vi "dc voltmeter.vi"() -> ()   [LabVIEW 2015]
panel:
  out "Color Indicator":u32(colorbox)
  out "String":string
  in  "Voltage":dbl
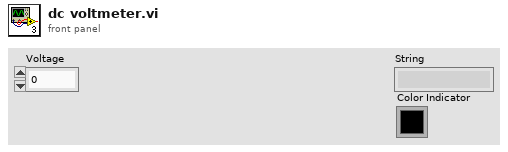
[diagram p1: front panel]
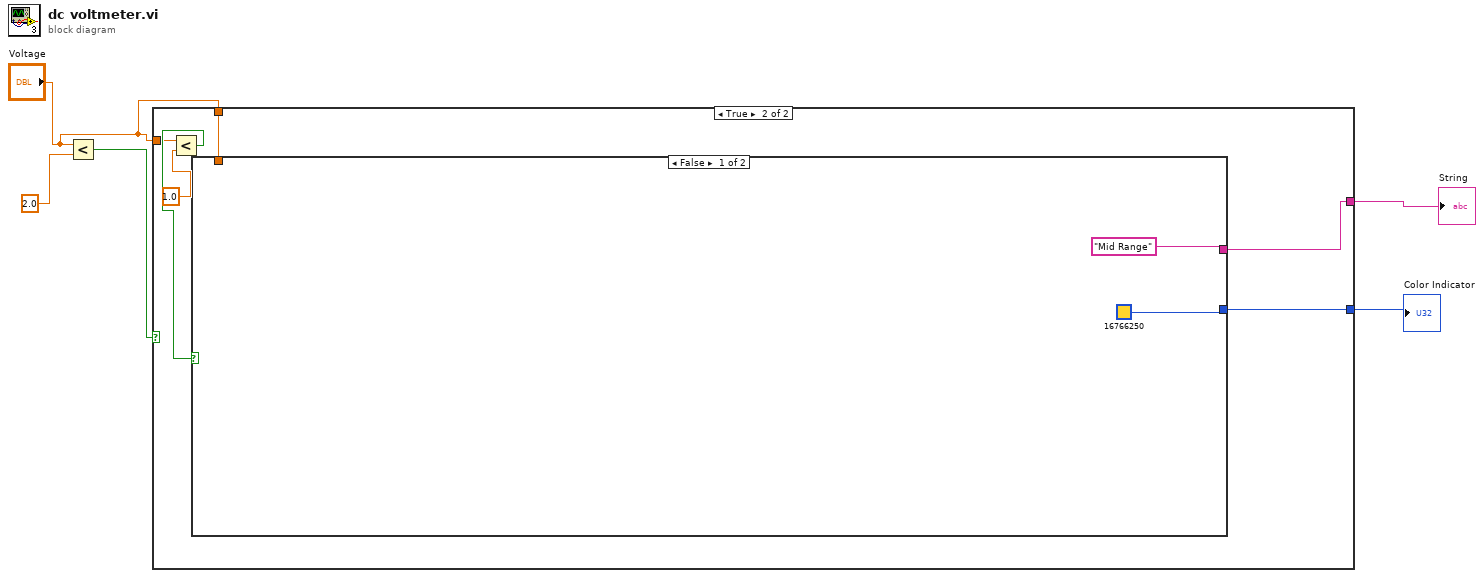
[diagram p0: block diagram]
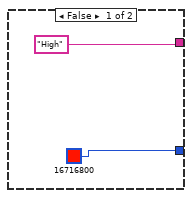
[diagram p2: hidden frame]
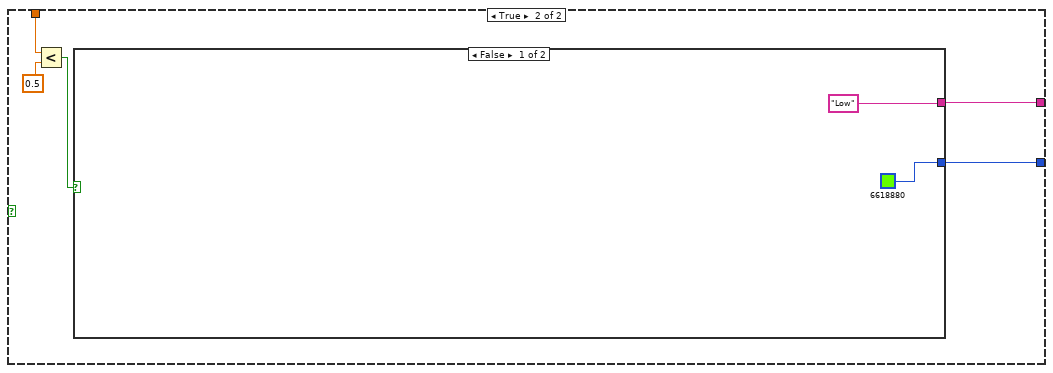
[diagram p3: hidden frame]
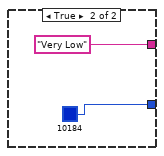
[diagram p4: hidden frame]
diagram:
  n1 = Less?(x="Voltage", y=2.0) -> (x < y?=w4:bool)
  n2 = case shown="True" w4 {
    tunnel: ["High" w11] -> w2
    tunnel: [u32 16716800 ("Color Box") w10] -> w3
    tunnel: "Voltage" -> [_ w9]
    tunnel: "Voltage" -> [_ w8]
    frame False {
    }
    frame True {
      n3 = Less?(x=w9, y=1.0) -> (x < y?=w12:bool)
      n4 = case shown="False" w12 {
        tunnel: ["Mid Range" w20] -> w11
        tunnel: [u32 16766250 ("Color Box") w19] -> w10
        tunnel: w8 -> [_ w18]
        frame False {
        }
        frame True {
          n5 = Less?(x=w18, y=0.5) -> (x < y?=w16:bool)
          n6 = case shown="False" w16 {
            tunnel: ["Low" "Very Low"] -> w20
            tunnel: [u32 6618880 ("Color Box") u32 10184 ("Color Box")] -> w19
            frame False {
            }
            frame True {
            }
          }
        }
      }
    }
  }
  "String" <- w2
  "Color Indicator" <- w3
